vi "校准数据选择表.vi"(11 "condition":string="where 测量模式=\"跨度核查\" and 数据标识 =\"N\" order by 时间 desc") -> (2 "布尔":bool=TRUE, 3 "ItemNames":string[](array[string]))   [LabVIEW 2016]
uses:
  <vilib>/Utility/miscctls.llb/LVPointTypeDef.ctl
panel:
  in  "确定":bool
  in  "返回":bool
  in  "数据表":T1
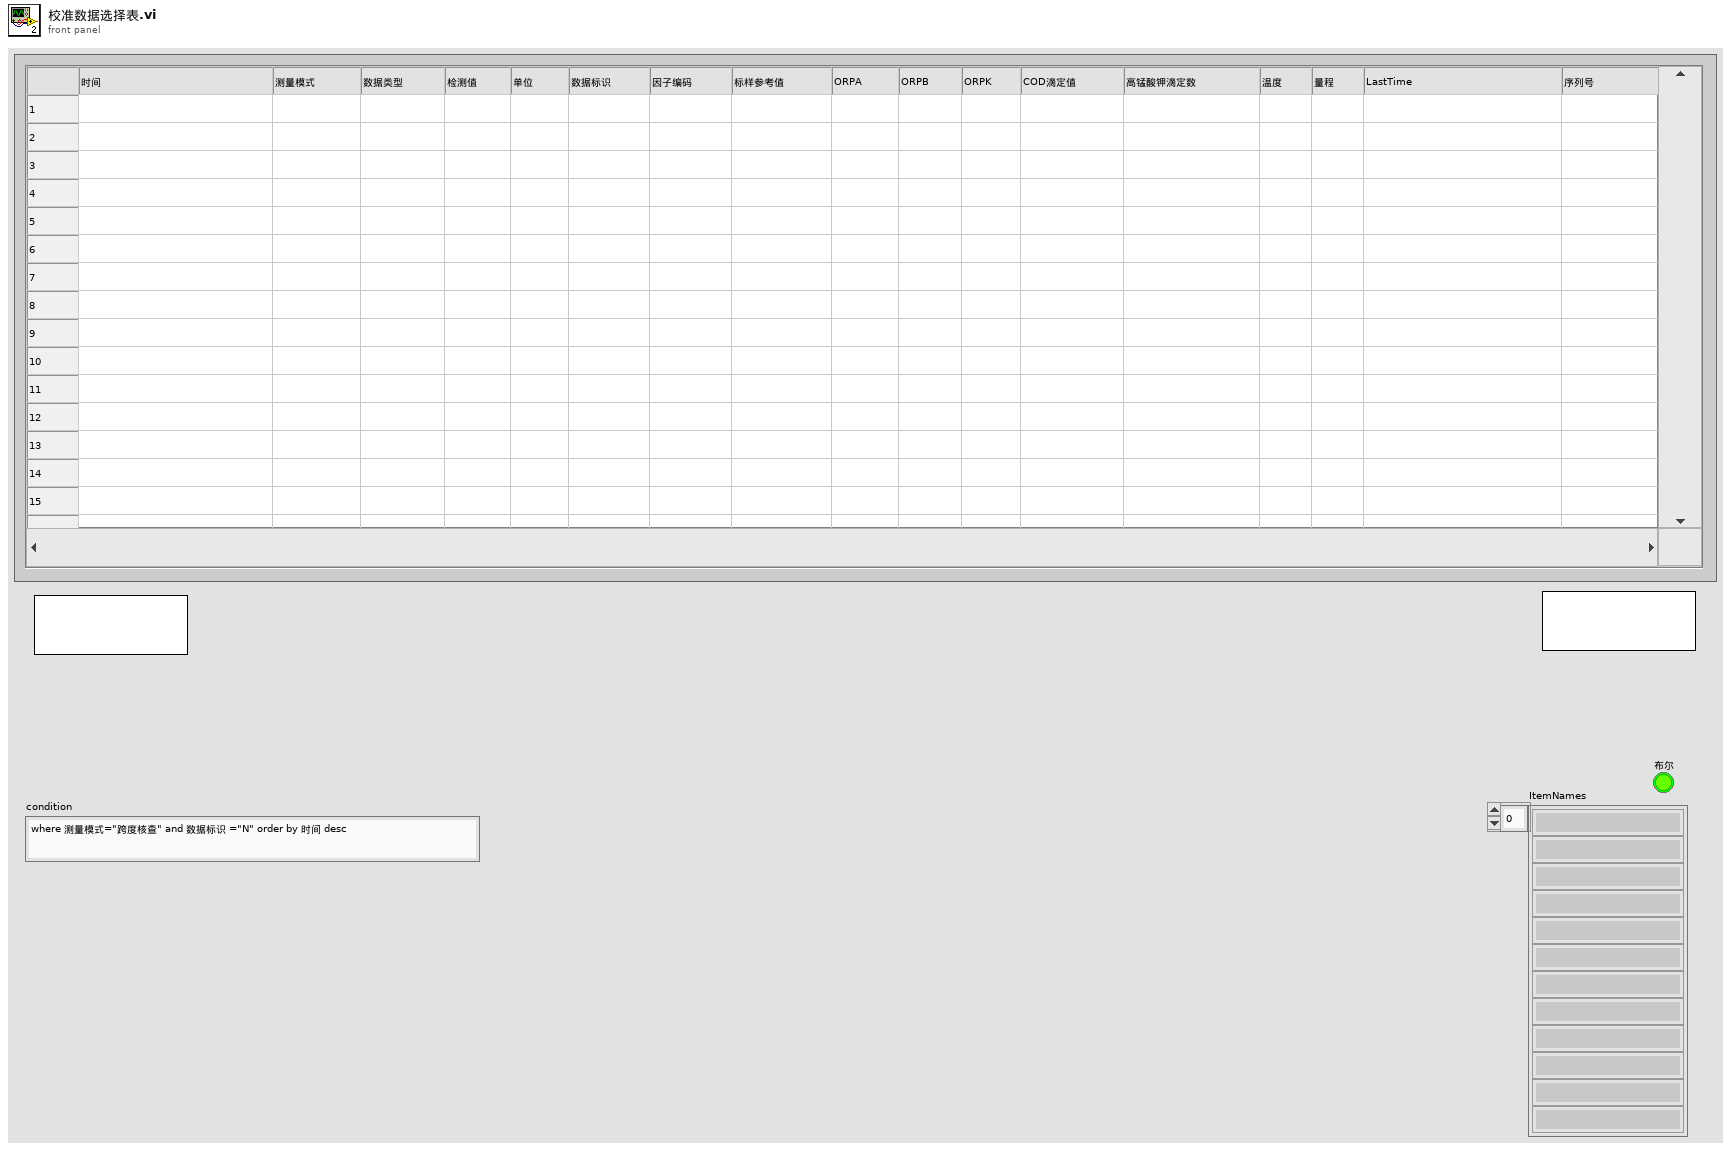
[diagram p1: front panel]
types:
  T1 = typedef "数据查询大列表框.ctl" = i32
  T2 = typedef "LVPointTypeDef.ctl" = cluster{"Horizontal":i16, "Vertical":i16}
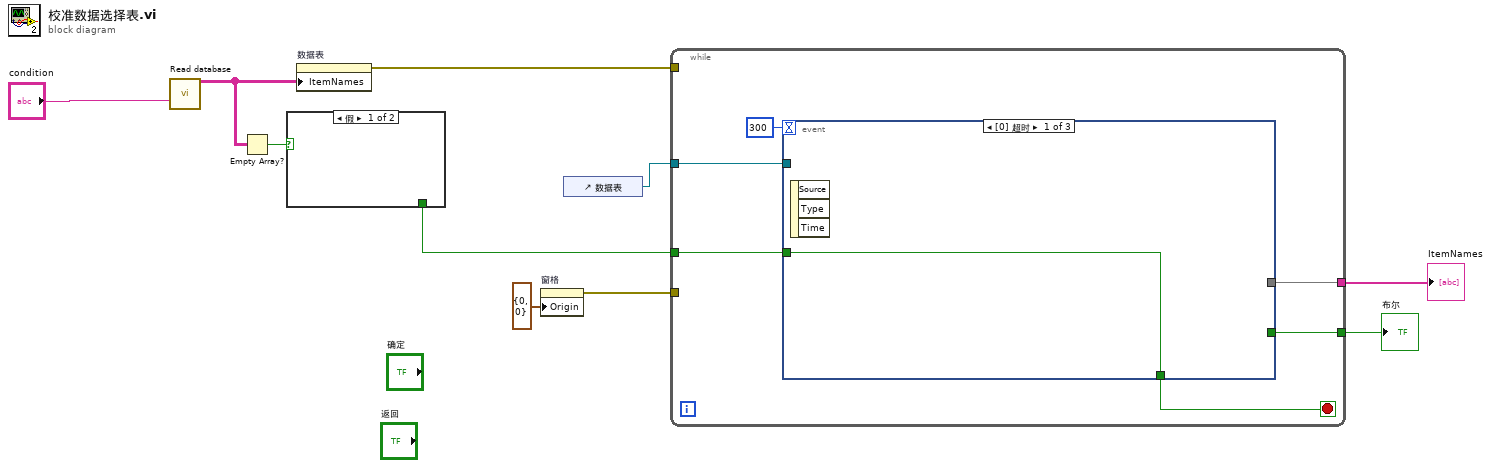
[diagram p0: block diagram]
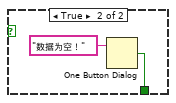
[diagram p2: hidden frame]
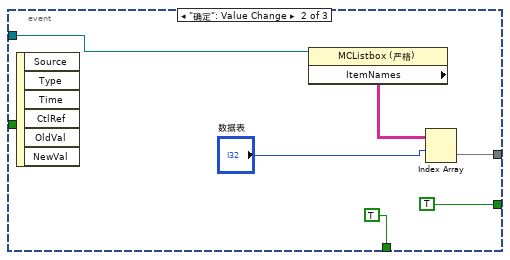
[diagram p3: hidden frame]
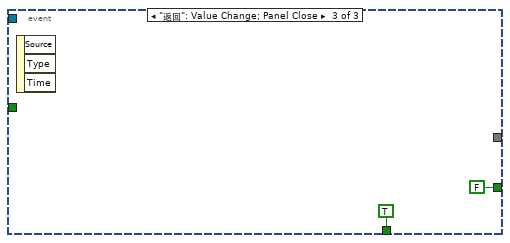
[diagram p4: hidden frame]
diagram:
  n1 = call "Read database.vi"("condition"="condition") -> ("表格"=w3:string[][])  [unwired: 9 in, 5 out]
  n2 = Empty Array?(array=w3) -> (empty?=w2:bool)
  n3 = case shown="假" w2 {
    tunnel: [_ w11] -> w1
    frame False {
    }
    frame True {
      n4 = One Button Dialog(message="数据为空！" ("消息")) -> (true=w11:bool)  [unwired: 1 in]
    }
  }
  n5 = property on="数据表" class="MCListbox (严格)"("ItemNames"=w3) -> (error out=w4:errorcluster)  [unwired: 2 in, 1 out]
  n6 = property on="窗格" class="Pane"("Origin"=T2 {"Horizontal"=0, "Vertical"=0} ("原点")) -> (error out=w6:errorcluster)  [unwired: 2 in, 1 out]
  n7 = control-ref of="数据表"() -> (w10:refnum<vi>)
  n8 = while {
    tunnel: w10 -> [w17]
    tunnel: [w16] -> w8
    tunnel: w6 -> [_]
    tunnel: [w15] -> w5
    tunnel: w4 -> [_]
    tunnel: w1 -> [w14]
    stop <- w18 stop-if-true
    n9 = event shown="[0] 超时" {
      selector: _ -> [_ _ _]
      dyn-events: _ -> [_ _ _]
      timeout: 300 -> [_ _ _]
      tunnel: [w19 TRUE TRUE] -> w18
      tunnel: w17 -> [_ w22 _]
      tunnel: [_ w23 _] -> w16
      tunnel: [_ TRUE FALSE] -> w15
      tunnel: w14 -> [w19 _ _]
      event Timeout {
        n10 = event-data() -> ()  [unwired: 1 in, 3 out]
      }
      event "确定": Value Change {
        n11 = event-data() -> ()  [unwired: 1 in, 6 out]
        n12 = property class="MCListbox (严格)"(reference=w22) -> ("ItemNames"=w24:string[][])  [unwired: 1 in, 2 out]
        n13 = Index Array(array=w24, index (row)="数据表") -> (element=w23:string[])  [unwired: 1 in]
      }
      event "返回": Value Change; Panel Close {
        n14 = event-data() -> ()  [unwired: 1 in, 3 out]
      }
    }
  }
  "ItemNames" <- w8
  "布尔" <- w5
